vi "FlatToRichpumploop_SystemInfo.vi"(5 "OutputClusterType":T1, 11 "InputCluster":T2) -> (3 "OutputCluster":T1)   [LabVIEW 2024, in "pumploop_client.lvlib"]
uses:
  pumploop_client.lvlib
  pumploop_SystemInfo_Flat.ctl
  pumploop_SystemInfo.ctl
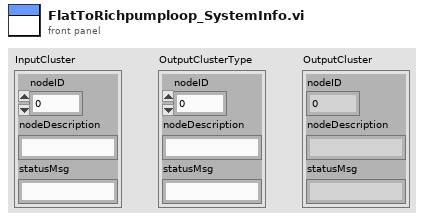
[diagram p1: front panel]
types:
  T1 = typedef "pumploop_client.lvlib/pumploop_SystemInfo.ctl" = cluster{"nodeID":i32, "nodeDescription":string, "statusMsg":string}
  T2 = typedef "pumploop_client.lvlib/pumploop_SystemInfo_Flat.ctl" = cluster{"nodeID":i32, "nodeDescription":string, "statusMsg":string}
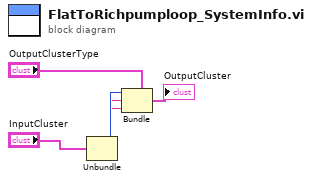
[diagram p0: block diagram]
diagram:
  n1 = Unbundle "Unbundle"("InputCluster") -> ("nodeID"=w3:i32, "nodeDescription"=w2:string, "statusMsg"=w1:string)
  n2 = Bundle "Bundle"(cluster="OutputClusterType", "nodeID"=w3, "nodeDescription"=w2, "statusMsg"=w1) -> (→"OutputCluster":T1)
